vi "Delete Impulse.vi"(1 "Impulse Direction +ve?":bool, 3 "Number of Impulses":i32, 4 "Impulse Plane":T2(ring), 5 "Impulse Positions (in)":T1(array[cluster]) {"Amplitude offset" format="%.2f"}, 9 "Plot Number":i32) -> (19 "Impulse Positions (out)":T1(array[cluster]) {"Amplitude offset" format="%.2f"})   [LabVIEW 2016, in "impulse functions.lvlib"]
uses:
  impulse functions.lvlib
panel:
  # "Copyright Americo A. Migliaccio (c) 2002 All Rights Reserved by Author"
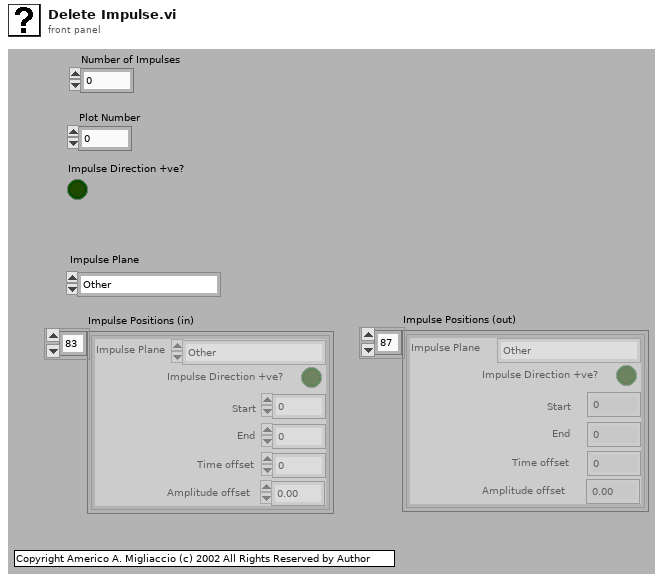
[diagram p1: front panel]
types:
  T1 = cluster{"Start":i32, "End":i32, "Impulse Plane":enum16{"Other", "Yaw", "Pitch", "Roll", "LARP", "RALP"}, "Impulse Direction +ve?":bool, "Time offset":i32, "Amplitude offset":dbl}[]
  T2 = enum16{"Other", "Yaw", "Pitch", "Roll", "LARP", "RALP"}
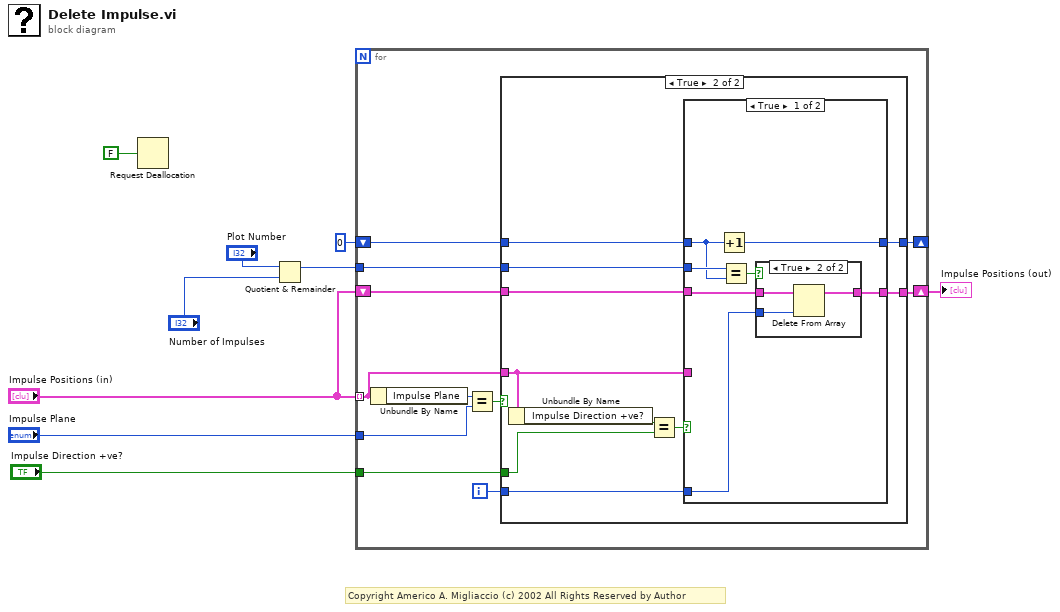
[diagram p0: block diagram]
diagram:
  # "Copyright Americo A. Migliaccio (c) 2002 All Rights Reserved by Author"
  n1 = Request Deallocation(FALSE ("flag")) -> ()
  n2 = Quotient & Remainder(x="Plot Number", y="Number of Impulses") -> (x-y*floor(x/y)=w2:i32)  [unwired: 1 out]
  n3 = for {
    tunnel: "Impulse Positions (in)" -> [w17] mode=indexing
    tunnel: "Impulse Plane" -> [w19]
    tunnel: "Impulse Direction +ve?" -> [w16]
    shift-right: [w12] -> _
    shift-left: 0 -> [w13]
    tunnel: w2 -> [w15]
    shift-right: [w10] -> w5
    shift-left: "Impulse Positions (in)" -> [w11]
    i -> [w14]
    n4 = Unbundle By Name(w17) -> ("Impulse Plane"=w20:T2)
    n5 = Equal?(x=w20, y=w19) -> (x = y?=w18:bool)
    n6 = case shown="True" w18 {
      tunnel: w17 -> [_ w32]
      tunnel: w16 -> [_ w31]
      tunnel: w15 -> [_ w28]
      tunnel: w14 -> [_ w26]
      tunnel: w11 -> [w21 w27]
      tunnel: w13 -> [w22 w25]
      tunnel: [w22 w24] -> w12
      tunnel: [w21 w23] -> w10
      frame False {
      }
      frame True {
        n7 = Unbundle By Name(w32) -> ("Impulse Direction +ve?"=w29:bool)
        n8 = Equal?(x=w29, y=w31) -> (x = y?=w30:bool)
        n9 = case shown="True" w30 {
          tunnel: w32 -> [_ _]
          tunnel: w28 -> [w39 _]
          tunnel: w26 -> [w37 _]
          tunnel: w27 -> [w38 w44]
          tunnel: w25 -> [w35 w45]
          tunnel: [w36 w45] -> w24
          tunnel: [w33 w44] -> w23
          frame True {
            n10 = Increment(x=w35) -> (x+1=w36:i32)
            n11 = Equal?(x=w39, y=w35) -> (x = y?=w34:bool)
            n12 = case shown="True" w34 {
              tunnel: w38 -> [w40 w43]
              tunnel: w37 -> [_ w42]
              tunnel: [w40 w41] -> w33
              frame False {
              }
              frame True {
                n13 = Delete From Array(array=w43, index=w42) -> (array with subset deleted=w41:T1)  [unwired: 1 in, 1 out]
              }
            }
          }
          frame False {
          }
        }
      }
    }
  }
  "Impulse Positions (out)" <- w5
